vi "编码输出.vi"(8 "error in (no error)":errorcluster, 11 "SingleStepTestV3输入":refnum<class "SingleStepTestV3.lvclass">) -> (0 "error out":errorcluster, 3 "SingleStepTestV3输出":refnum<class "SingleStepTestV3.lvclass">)   [LabVIEW 2022 SP3, in "SingleStepTestV3.lvlib" / "SingleStepTestV3.lvclass"]
uses:
  SingleStepTestV3.lvclass
  SingleStepTestV3.lvclass/SingleStepTestV3.ctl
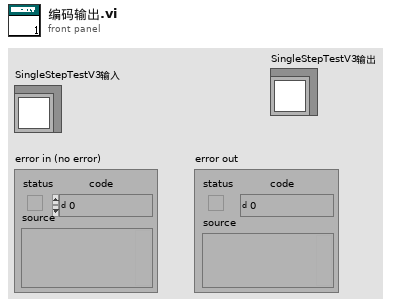
[diagram p1: front panel]
types:
  T1 = typedef "SingleStepTestV3.lvlib/SingleStepTestV3.lvclass/State Data.ctl" = cluster{"data":u16[], "仪器版本":T2}
  T2 = typedef "SingleStepTestV3.lvlib/SingleStepTestV3.lvclass/仪器版本.ctl" = enum16{"V3.1版", "V4版", "V3版", "V4.2版"}
  T3 = typedef "SingleStepTestV3.lvclass/注射泵操作.ctl" = enum32{"复位", "注入", "注出", "等待"}
  T4 = typedef "SingleStepTestV3.lvclass/阀口操作.ctl" = enum32{"未选择", "V1", "V2", "V3", "V4", "V5", "V6", "V7", "V8", "V9", "V10", "V11", "V12"}
  T5 = typedef "SingleStepTestV3.lvclass/灯选择.ctl" = enum32{"未选择", "365", "520", "660", "氙灯/紫灯"}
  T6 = typedef "SingleStepTestV3.lvclass/ADC选择.ctl" = enum32{"未选择", "ADC365", "ADC520", "ADC660", "光谱仪"}
  T7 = typedef "SingleStepTestV3.lvclass/外设选择2.ctl" = cluster{"V9-1":bool, "V9-2":bool, "顺时针":bool, "逆时针":bool}
  T8 = typedef "SingleStepTestV3.lvclass/控温操作.ctl" = cluster{"氨氮控温":bool, "消解":bool, "恒温":bool, "降温":bool}
  T9 = typedef "SingleStepTestV3.lvclass/外设选择.ctl" = cluster{"蠕动泵":bool, "电磁阀1":bool, "电磁阀2":bool, "慢速":bool}
  T10 = typedef "SingleStepTestV3.lvlib/SingleStepTestV3.lvclass/ADC选择2.ctl" = bool
  T11 = typedef "SingleStepTestV3.lvclass/项目输入.ctl" = u16
  T12 = typedef "SingleStepTestV3.lvclass/数值输入.ctl" = i16
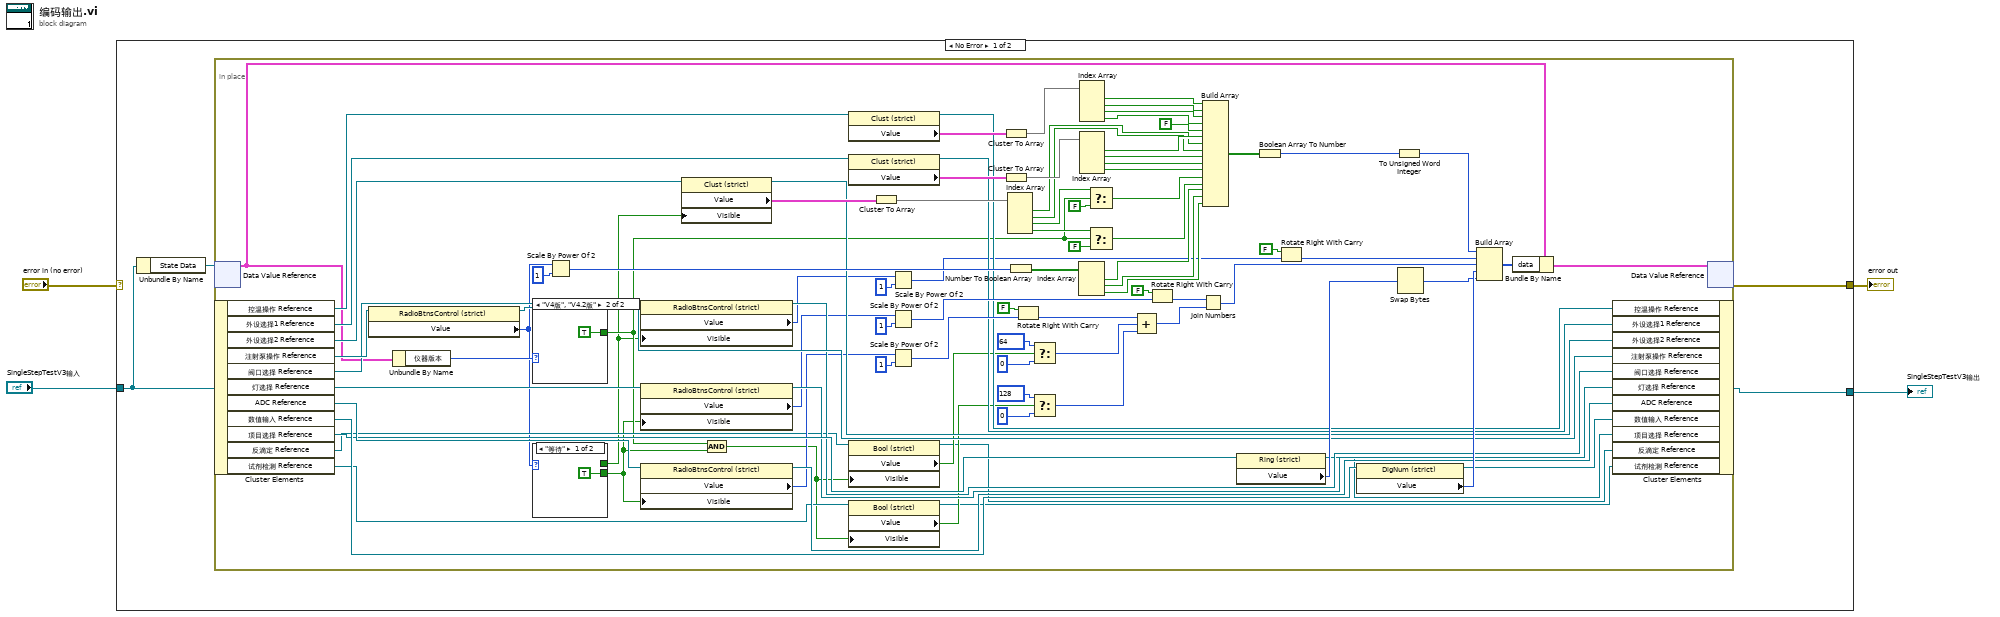
[diagram p0: block diagram]
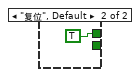
[diagram p2: hidden frame]
diagram:
  n1 = case shown="No Error" "error in (no error)" {
    selector: "error in (no error)" -> [_ w104]
    tunnel: "SingleStepTestV3输入" -> [w7 w103]
    tunnel: [w6 w104] -> w3
    tunnel: [w5 w103] -> w1
    frame No Error {
      n2 = Unbundle By Name(w7) -> ("State Data"=w8:refnum<data-value>)
      n3 = in-place {
        n4 = in-place-dvr #1(w8) -> (w38:T1)  [unwired: 1 out]
        n5 = in-place-cluster #2(w7) -> ("控温操作 Reference"=w99:refnum<vi>, "外设选择1 Reference"=w84:refnum<vi>, "外设选择2 Reference"=w83:refnum<vi>, "注射泵操作 Reference"=w82:refnum<vi>, "阀口选择 Reference"=w72:refnum<vi>, "灯选择 Reference"=w70:refnum<vi>, "ADC Reference"=w69:refnum<vi>, "数值输入 Reference"=w66:refnum<vi>, "项目选择 Reference"=w65:refnum<vi>, "反滴定 Reference"=w27:refnum<vi>, "试剂检测 Reference"=w26:refnum<vi>)
        n6 = property class="RadioBtnsControl (strict)"(reference=w82) -> (reference out=w52:refnum<vi>, "Value"=w13:T3)  [unwired: 1 in, 1 out]
        n7 = Unbundle By Name(w38) -> ("仪器版本"=w28:T2)
        n8 = case shown="\"V4版\", \"V4.2版\"" w28 {
          tunnel: [_ TRUE] -> w11
          frame "V3.1版", Default {
          }
          frame "V4版", "V4.2版" {
          }
        }
        n9 = case shown="\"等待\"" w13 {
          tunnel: [TRUE _] -> w10
          tunnel: [_ TRUE] -> w9
          frame "等待" {
          }
          frame "复位", Default {
          }
        }
        n10 = Scale By Power Of 2(n=w13, x=u8 1) -> (x*2^n=w94:u8)
        n11 = property class="RadioBtnsControl (strict)"(reference=w72, "Visible"=w9) -> (reference out=w51:refnum<vi>, "Value"=w44:T4)  [unwired: 1 in, 1 out]
        n12 = property class="RadioBtnsControl (strict)"(reference=w70, "Visible"=w10) -> (reference out=w50:refnum<vi>, "Value"=w39:T5)  [unwired: 1 in, 1 out]
        n13 = property class="RadioBtnsControl (strict)"(reference=w69, "Visible"=w10) -> (reference out=w49:refnum<vi>, "Value"=w40:T6)  [unwired: 1 in, 1 out]
        n14 = property class="Clust (strict)"(reference=w83, "Visible"=w9) -> (reference out=w53:refnum<vi>, "Value"=w96:T7)  [unwired: 1 in, 1 out]
        n15 = And(x=w11, y=w10) -> (x .and. y?=w12:bool)
        n16 = property class="Clust (strict)"(reference=w99) -> (reference out=w55:refnum<vi>, "Value"=w98:T8)  [unwired: 1 in, 1 out]
        n17 = property class="Clust (strict)"(reference=w84) -> (reference out=w54:refnum<vi>, "Value"=w97:T9)  [unwired: 1 in, 1 out]
        n18 = property class="Bool (strict)"(reference=w27, "Visible"=w12) -> (reference out=w15:refnum<vi>, "Value"=w25:T10)  [unwired: 1 in, 1 out]
        n19 = property class="Bool (strict)"(reference=w26, "Visible"=w12) -> (reference out=w14:refnum<vi>, "Value"=w20:T10)  [unwired: 1 in, 1 out]
        n20 = Cluster To Array(cluster=w96) -> (array=w92:bool[])
        n21 = Scale By Power Of 2(n=w44, x=u16 1) -> (x*2^n=w29:u16)
        n22 = Scale By Power Of 2(n=w39, x=u8 1) -> (x*2^n=w62:u8)
        n23 = Scale By Power Of 2(n=w40, x=u8 1) -> (x*2^n=w63:u8)
        n24 = Cluster To Array(cluster=w98) -> (array=w90:bool[])
        n25 = Cluster To Array(cluster=w97) -> (array=w91:bool[])
        n26 = Index Array(array=w92) -> (element #1=w77:bool, element #2=w76:bool, element #3=w37:bool, element #4=w34:bool)  [unwired: 4 in]
        n27 = Number To Boolean Array(number=w94) -> (Boolean array=w93:bool[])
        n28 = Rotate Right With Carry(2:w63, 3:FALSE ("进位")) -> (0:w17:u8)  [unwired: 1 out]
        n29 = Select(t=u8 64 ("x"), s=w25, f=u8 0 ("x")) -> (s? t:f=w19:u8)
        n30 = Select(t=u8 128 ("x"), s=w20, f=u8 0 ("x")) -> (s? t:f=w18:u8)
        n31 = Index Array(array=w93) -> (element #1=w75:bool, element #2=w74:bool, element #3=w73:bool)  [unwired: 3 in]
        n32 = Index Array(array=w90) -> (element #1=w89:bool, element #2=w88:bool, element #3=w87:bool, element #4=w86:bool)  [unwired: 4 in]
        n33 = Index Array(array=w91) -> (element #1=w81:bool, element #2=w80:bool, element #3=w79:bool, element #4=w78:bool)  [unwired: 4 in]
        n34 = Select(t=w37, s=w11, f=FALSE) -> (s? t:f=w36:bool)
        n35 = Select(t=w34, s=w11, f=FALSE) -> (s? t:f=w33:bool)
        n36 = Compound Arithmetic op=ADD(w17, w19, w18) -> (w16:u8)
        n37 = Rotate Right With Carry(2:w62, 3:FALSE ("进位")) -> (0:w43:u8)  [unwired: 1 out]
        n38 = Join Numbers(hi=w43, lo=w16) -> ((hi.lo)=w59:u16)
        n39 = Build Array(w89, w88, w87, w86, FALSE, w81, w77, w76, w80, w79, w78, w36, w33, w75, w74, w73) -> (w61:bool[])
        n40 = property class="Ring (strict)"(reference=w65) -> (reference out=w47:refnum<vi>, "Value"=w64:T11)  [unwired: 1 in, 1 out]
        n41 = Boolean Array To Number(Boolean array=w61) -> (number=w60:u32)
        n42 = Rotate Right With Carry(2:w29, 3:FALSE ("进位")) -> (0:w30:u16)  [unwired: 1 out]
        n43 = property class="DigNum (strict)"(reference=w66) -> (reference out=w48:refnum<vi>, "Value"=w58:T12)  [unwired: 1 in, 1 out]
        n44 = To Unsigned Word Integer(number=w60) -> (unsigned 16bit integer=w56:u16)
        n45 = Swap Bytes(anything=w64) -> (byte swapped=w57:T11)
        n46 = Build Array(w56, w30, w59, w58, w57) -> (w45:T11[])
        n47 = Bundle By Name(cluster=w38, "data"=w45) -> (w46:T1)
        n48 = in-place-cluster #2("控温操作 Reference"=w55, "外设选择1 Reference"=w54, "外设选择2 Reference"=w53, "注射泵操作 Reference"=w52, "阀口选择 Reference"=w51, "灯选择 Reference"=w50, "ADC Reference"=w49, "数值输入 Reference"=w48, "项目选择 Reference"=w47, "反滴定 Reference"=w15, "试剂检测 Reference"=w14) -> (w5:refnum<class "SingleStepTestV3.lvclass">)
        n49 = in-place-dvr #1(w46) -> (w6:errorcluster)  [unwired: 1 out]
      }
    }
    frame Error {
    }
  }
  "error out" <- w3
  "SingleStepTestV3输出" <- w1
